vi "Actor Core.vi"(8 "error in":errorcluster, 11 "Instrument in":refnum<class "Instrument.lvclass">) -> (0 "error out":errorcluster, 3 "Actor out":refnum<class "Actor.lvclass">)   [LabVIEW 2019, in "Instrument.lvlib" / "Instrument.lvclass"]
doc: "The user interface for this panel.\n\n----\nPlease see the following web address for additional documentation and tutorial information:\nhttp://www.mooregoodideas.com/mgi-panel-manager/\n\nAuthor: Derek Trepanier\n\nCopyright (c) 2018, Moore Good Ideas, Inc.\n\nAll rights reserved.\n\nRedistribution and use in source and binary forms, with or without modification, are permitted provided that the following conditions are met:\n\n * Redistributions of source code must retain the above copyright notice, this list of conditions and the following disclaimer.\n * Redistributions in binary form must reproduce the above copyright notice, this list of conditions and the following disclaimer in the documentation and/or other materials provided with the distribution.\n * Neither the name of Moore Good Ideas, Inc. nor the names of its contributors may be used to endorse or promote products derived from this software without specific prior written permission.\n\nTHIS SOFTWARE IS PROVIDED BY THE COPYRIGHT HOLDERS AND CONTRIBUTORS \"AS IS\" AND ANY EXPRESS OR IMPLIED WARRANTIES, INCLUDING, BUT NOT LIMITED TO, THE IMPLIED WARRANTIES OF MERCHANTABILITY AND FITNESS FOR A PARTICULAR PURPOSE ARE DISCLAIMED. IN NO EVENT SHALL THE COPYRIGHT OWNER OR CONTRIBUTORS BE LIABLE FOR ANY DIRECT, INDIRECT, INCIDENTAL, SPECIAL, EXEMPLARY, OR CONSEQUENTIAL DAMAGES (INCLUDING, BUT NOT LIMITED TO, PROCUREMENT OF SUBSTITUTE GOODS OR SERVICES; LOSS OF USE, DATA, OR PROFITS; OR BUSINESS INTERRUPTION) HOWEVER CAUSED AND ON ANY THEORY OF LIABILITY, WHETHER IN CONTRACT, STRICT LIABILITY, OR TORT (INCLUDING NEGLIGENCE OR OTHERWISE) ARISING IN ANY WAY OUT OF THE USE OF THIS SOFTWARE, EVEN IF ADVISED OF THE POSSIBILITY OF SUCH DAMAGE."
uses:
  Instrument.lvclass
  C:/Program Files (x86)/National Instruments/LabVIEW 2019/vi.lib/MGI/Panel Manager/Panel Actor/Panel Actor/Panel Actor.lvclass
  <vilib>/ActorFramework/Actor/Actor.lvclass
  <vilib>/ActorFramework/Message Enqueuer/Message Enqueuer.lvclass/Message Enqueuer.ctl
  <vilib>/ActorFramework/Message Enqueuer/Enqueue.vi
  <vilib>/MGI/Panel Manager/Panel/Panel/Subpanel/Subpanel.lvclass
  C:/Program Files (x86)/National Instruments/LabVIEW 2019/vi.lib/MGI/Panel Manager/Panel/Panel/Panel.lvclass
  <vilib>/ActorFramework/Stop Msg/Stop Msg.lvclass
  C:/Program Files (x86)/National Instruments/LabVIEW 2019/vi.lib/ActorFramework/Message/Message.lvclass
  <vilib>/MGI/Panel Manager/Panel/Panel/Subpanel/Subpanel.vi
  <vilib>/ActorFramework/Message Priority Queue/Priority Enqueue.vi
  <vilib>/MGI/Panel Manager/Panel Actor/Panel Actor/Panel Actor.lvclass
  <vilib>/MGI/Panel Manager/Panel/Panel.lvlib
panel:
  out "Title":string
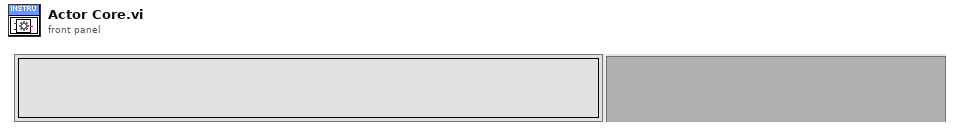
[diagram p1: front panel]
types:
  T1 = enum32{"Invalid", "Standard", "Closed", "Hidden", "Minimized", "Maximized"}
  T2 = enum8{"Enabled", "Disabled", "Disabled and Grayed Out"}
  T3 = typedef "Panel.lvlib/Panel Helper.lvclass/Events.ctl" = enum16{"Initialized", "Shown", "Hidden", "Closed"}
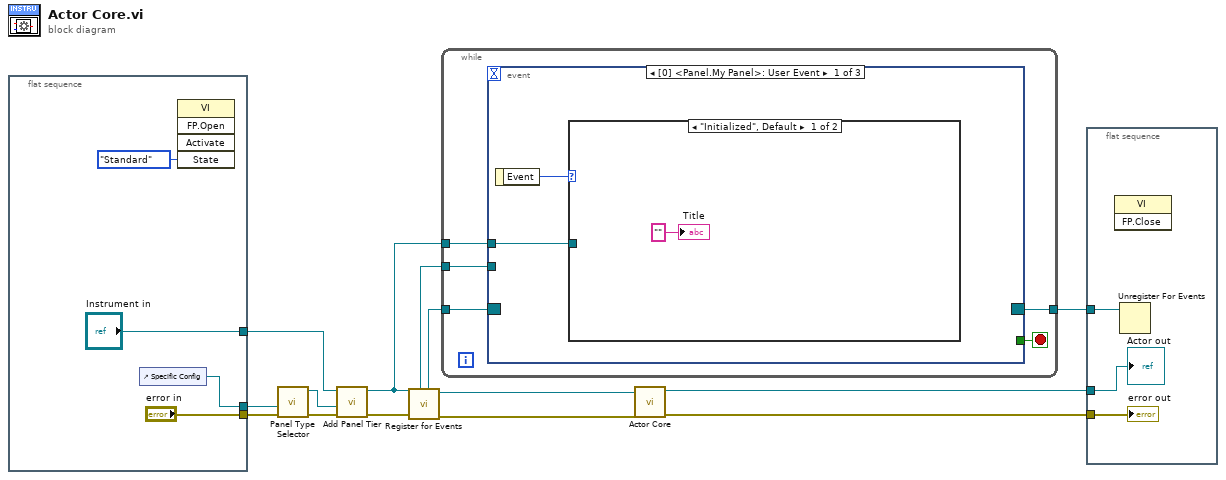
[diagram p0: block diagram]
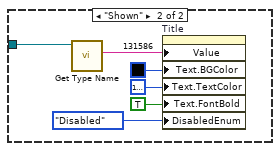
[diagram p2: hidden frame]
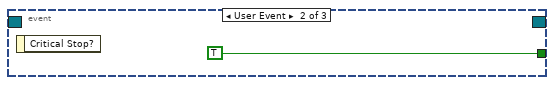
[diagram p3: hidden frame]
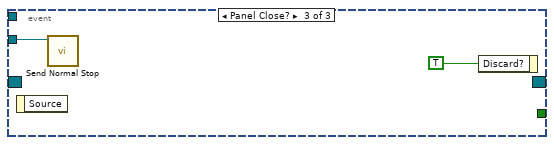
[diagram p4: hidden frame]
diagram:
  n1 = flat-sequence {
    tunnel: ["error in"] -> w14
    tunnel: ["Instrument in"] -> w9
    tunnel: [w17] -> w11
    frame #0 {
      n2 = control-ref of="Specific Config"() -> (w17:refnum<vi>)
      n3 = invoke class="VI" method="FP.Open"("State"=T1."Standard") -> ()  [unwired: 4 in, 5 out]
    }
  }
  n4 = call-poly <vilib>:"Panel Type Selector.vi"("Error In"=w14, "Sub Panel"=w11) -> ("Error Out"=w10:errorcluster, "Subpanel Out"=w13:refnum<class "Subpanel.lvclass">)  [unwired: 8 in]
  n5 = call <vilib>:"Add Panel Tier.vi"("Error In"=w10, "Old VI's Destination"=w13, "Panel Actor in"=w9) -> ("Error Out"=w7:errorcluster, "Panel Actor out"=w1:refnum<class "Instrument.lvclass">)  [unwired: 7 in]
  n6 = call <vilib>:"Register for Events.vi"("Error In"=w7, "Panel Actor in"=w1) -> ("Error Out"=w4:errorcluster, "Panel Actor out"=w3:refnum<class "Instrument.lvclass">, "Pnl Actor"=w5:refnum<event-registration>, "Self Enqueuer"=w6:refnum<class "Message Enqueuer.lvclass">)  [unwired: 6 in]
  n7 = while {
    tunnel: w5 -> [w23]
    tunnel: w6 -> [w22]
    tunnel: [w20] -> w2
    tunnel: w1 -> [w19]
    stop <- w21 stop-if-true
    n8 = event shown="[0] <Panel.My Panel>: User Event" {
      selector: w23 -> [_ _ _]
      dyn-events: [_ _ _] -> w20
      timeout: _ -> [_ _ _]
      tunnel: w22 -> [_ _ w35]
      tunnel: [_ TRUE _] -> w21
      tunnel: w19 -> [w24 _ _]
      event User Event {
        n9 = event-data() -> ("Event"=w25:T3)  [unwired: 1 in]
        n10 = case shown="\"Initialized\", Default" w25 {
          tunnel: w24 -> [_ w27]
          frame "Initialized", Default {
            "Title" <- "" ("Heads")
          }
          frame "Shown" {
            n11 = call-dynamic "Get Type Name.vi"("Instrument in"=w27) -> ("Type Name"=w32:string)  [unwired: 10 in]
            n12 = property on="Title" class="Str"("Value"=w32, "Text.BGColor"=u32 131586 ("Text.Text Colors:BG Color"), "Text.TextColor"=u32 16777225 ("Text.Text Colors:Text Color"), "Text.FontBold"=TRUE ("Text.Font:Bold"), "DisabledEnum"=T2."Disabled" ("Disabled")) -> ()  [unwired: 2 in, 2 out]
          }
        }
      }
      event User Event {
        n13 = event-data() -> ()  [unwired: 1 in, 1 out]
      }
      event Panel Close? {
        n14 = event-data() -> ()  [unwired: 1 in, 1 out]
        n15 = call <vilib>:"Send Normal Stop.vi"("Message Enqueuer"=w35) -> ()  [unwired: 10 in, 1 out]
        n16 = event-data("Discard?"=TRUE) -> ()  [unwired: 1 in, 1 out]
      }
    }
  }
  n17 = call-parent "Actor Core.vi"("error in"=w4, "Panel Actor in"=w3) -> ("error out"=w8:errorcluster, "Actor out"=w12:refnum<class "Actor.lvclass">)  [unwired: 8 in]
  n18 = flat-sequence {
    tunnel: w12 -> [w38]
    tunnel: w8 -> [w37]
    tunnel: w2 -> [w36]
    frame #0 {
      n19 = invoke class="VI" method="FP.Close"() -> ()  [unwired: 3 in, 3 out]
      n20 = Unregister For Events(event registration refnum=w36) -> ()  [unwired: 1 in, 1 out]
      "error out" <- w37
      "Actor out" <- w38
    }
  }
